vi "Chart Round to Nearest Integer.vi"() -> ()   [LabVIEW 2019]
panel:
  out "Chart":dbl(graph)
  in  "Push this button to stop the program":bool
  in  "Input numbers using the slide":dbl(slide) scale=0.0..10.0
  # "Challenge: Write a program that takes numbers entered via a slide and rounds each one to the nearest integer, displayingf the results on a scrolling chart."
  # "Try it: Run the program and use the slide to input numbers."
  # "You will probably need:\nControls, waveform chart, wait for ms, numeric functions."
  # "Open the block diagram to see a possible solution."
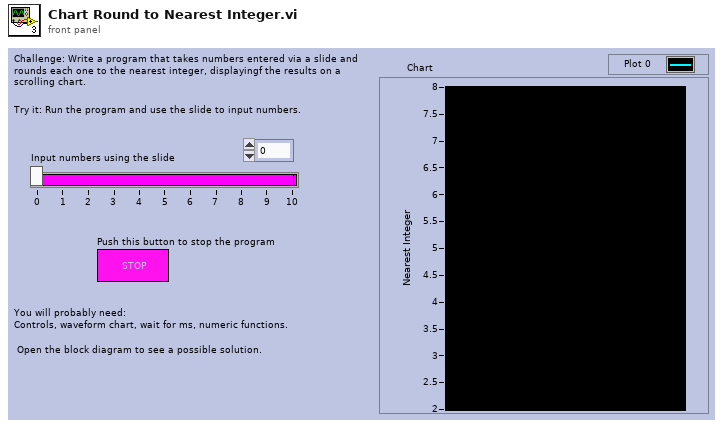
[diagram p1: front panel]
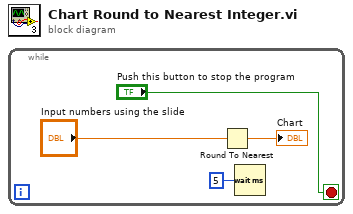
[diagram p0: block diagram]
diagram:
  n1 = while {
    stop <- "Push this button to stop the program" stop-if-true
    n2 = Round To Nearest(number="Input numbers using the slide") -> (nearest integer value=→"Chart":dbl)
    n3 = Wait (ms)(milliseconds to wait=u32 5) -> ()  [unwired: 1 out]
  }
